vi "DellItem.vi"(8 "Error":errorcluster, 10 "Tag":string[](array[string]), 11 "Tree in":refnum<class "Tree.lvclass">) -> (0 "Error":errorcluster, 1 "StepForward":T1(ring), 2 "StepBack":T1(ring), 3 "Tree out":refnum<class "Tree.lvclass">)   [LabVIEW 2021, in "Tree.lvlib" / "Tree.lvclass"]
uses:
  Tree.lvclass
  Private/TreeControllerTag.ctl
  Tree.lvclass/Tree.ctl
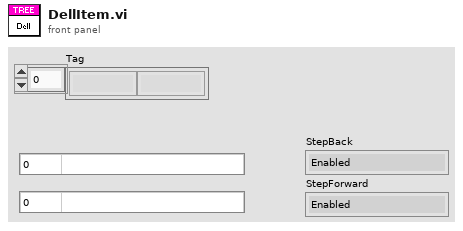
[diagram p1: front panel]
types:
  T1 = enum8{"Enabled", "Disabled", "Disabled and Grayed Out"}
  T2 = typedef "Tree.lvlib/Tree.lvclass/TreeControllerTag.ctl" = enum8{"Null", "1. Add item", "2. Delete item", "3. Get All Tree Data", "4. Drag Starting", "5. Drag Ended", "6. Add Tree Values", "7. Get Item Value", "8. Edit Item", "9. StepBack", "10. Filter"}
  T3 = cluster{"StepBack":enum8{"Enabled", "Disabled", "Disabled and Grayed Out"}, "StepForward":enum8{"Enabled", "Disabled", "Disabled and Grayed Out"}}
  T4 = cluster{"Tag":string[], "queue out":refnum<queue>}
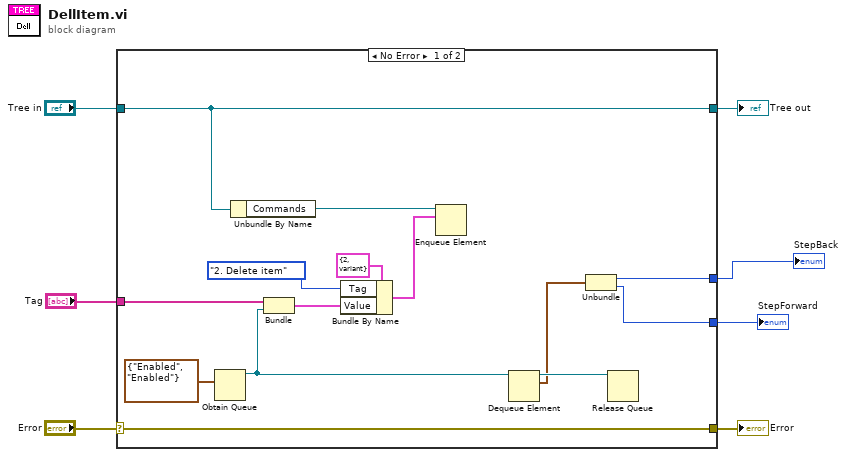
[diagram p0: block diagram]
diagram:
  n1 = case shown="No Error" "Error" {
    selector: "Error" -> [w21 w23]
    tunnel: [w21 w23] -> w6
    tunnel: [w20 w22] -> w4
    tunnel: "Tree in" -> [w20 w22]
    tunnel: "Tag" -> [w16 _]
    tunnel: [w10 _] -> w2
    tunnel: [w9 _] -> w1
    frame No Error {
      n2 = Obtain Queue(element data type=T3 {"StepBack"=enum."Enabled", "StepForward"=enum."Enabled"} ("output cluster")) -> (queue out=w14:refnum<queue>)  [unwired: 4 in, 2 out]
      n3 = Unbundle By Name(w20) -> ("Commands"=w19:refnum<queue>)
      n4 = Bundle("Tag"=w16, "queue out"=w14) -> (w12:T4)  [unwired: 1 in]
      n5 = Bundle By Name(cluster=cluster{"Tag":u8, "Value":variant} {"Tag"=2, "Value"=variant} ("element"), "Tag"=TreeControllerTag."2. Delete item", "Value"=w12) -> (w17:cluster{"Tag":u8, "Value":variant})
      n6 = Enqueue Element(queue=w19, element=w17) -> ()  [unwired: 2 in, 3 out]
      n7 = Dequeue Element(queue=w14) -> (queue out=w13:refnum<queue>, element=w11:T3)  [unwired: 2 in, 2 out]
      n8 = Unbundle(w11) -> ("StepBack"=w10:T1, "StepForward"=w9:T1)
      n9 = Release Queue(queue=w13) -> ()  [unwired: 2 in, 3 out]
    }
    frame Error {
    }
  }
  "Error" <- w6
  "Tree out" <- w4
  "StepBack" <- w2
  "StepForward" <- w1
